vi "Module Identities.vi"(8 "error in (no error)":errorcluster, 11 "PluginGUI in":refnum<class "PluginGUI.lvclass">) -> (0 "error out":errorcluster, 2 "Identities":refnum<class "Identity.lvclass">[](array[class]), 3 "PluginGUI out":refnum<class "PluginGUI.lvclass">)   [LabVIEW 2020, in "VolatusGUI.lvlib" / "PluginGUI.lvclass"]
uses:
  PluginGUI.lvclass
  Volatus/Identity/Identity.lvclass
  PluginGUI.lvclass/PluginGUI.ctl
  GUI Identity/GUI Identity.lvclass
  C:/dev/lv20CE/relink/lv-volatus/VolatusGUI/GUI Identity/GUI Identity.lvclass
  C:/dev/lv20CE/relink/lv-volatus/Volatus/Identity/Identity.lvclass
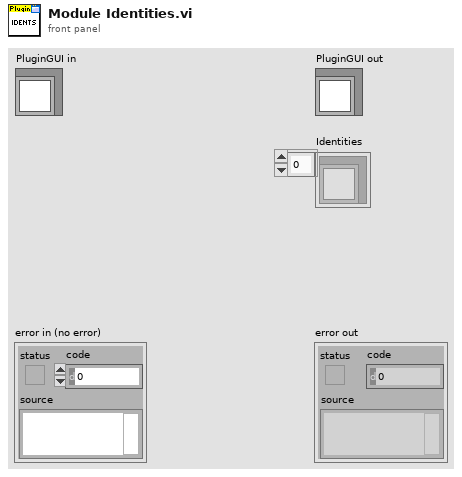
[diagram p1: front panel]
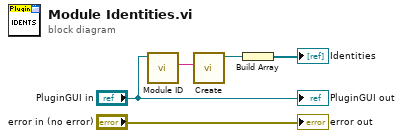
[diagram p0: block diagram]
diagram:
  n1 = call-dynamic "Module ID.vi"("Module in"="PluginGUI in") -> ("Module ID"=w3:string)  [unwired: 10 in]
  n2 = call "Create.vi"("Module ID"=w3) -> ("GUI Identity out"=w2:refnum<class "GUI Identity.lvclass">)  [unwired: 10 in]
  n3 = Build Array(w2) -> (→"Identities":refnum<class "GUI Identity.lvclass">[])
  "error out" <- "error in (no error)"
  "PluginGUI out" <- "PluginGUI in"
